vi "Encoder_Correction.vi"(6 "Left X":dbl, 9 "Left Y":dbl, 10 "Right Y":dbl) -> ()   [LabVIEW 2013]
panel:
  out "rr":dbl
  out "fr":dbl
  out "rl":dbl
  out "fl":dbl
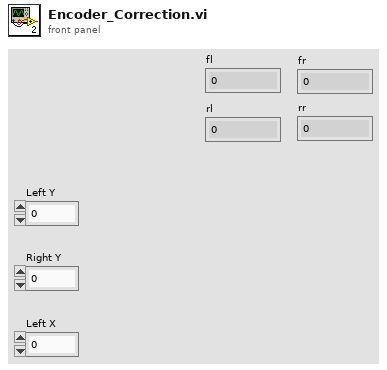
[diagram p1: front panel]
types:
  T1 = typedef "WPI_EncoderDevRef.ctl" = cluster{"DevStatus":errorcluster, "EncoderIndex":T2, "CounterIndex":T3, "DistancePerCount":dbl, "Decoding Type":T4}
  T2 = typedef "FPGA_EncoderIdx.ctl" = enum8{"Enc 0", "Enc 1", "Enc 2", "Enc 3", "Invalid"}
  T3 = typedef "FPGA_CounterCtrSystemIndex.ctl" = enum8{"Ctr 0", "Ctr 1", "Ctr 2", "Ctr 3", "Ctr 4", "Ctr 5", "Ctr 6", "Ctr 7", "Invalid"}
  T4 = typedef "WPI_EncoderType.ctl" = enum16{"1x", "2x", "4x"}
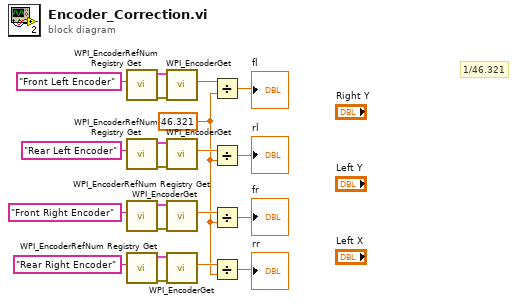
[diagram p0: block diagram]
diagram:
  w1 = 46.321 ("y")
  # "1/46.321"
  n1 = call <vilib>:"WPI_EncoderRefNum Registry Get.vi"("refnum name"="Front Left Encoder") -> ("error out"=w21:errorcluster, "EncoderDevRef"=w20:T1)  [unwired: 9 in]
  n2 = call <vilib>:"WPI_EncoderRefNum Registry Get.vi"("refnum name"="Rear Left Encoder") -> ("error out"=w18:errorcluster, "EncoderDevRef"=w17:T1)  [unwired: 9 in]
  n3 = call <vilib>:"WPI_EncoderRefNum Registry Get.vi"("refnum name"="Front Right Encoder") -> ("error out"=w15:errorcluster, "EncoderDevRef"=w14:T1)  [unwired: 9 in]
  n4 = call <vilib>:"WPI_EncoderRefNum Registry Get.vi"("refnum name"="Rear Right Encoder") -> ("error out"=w12:errorcluster, "EncoderDevRef"=w11:T1)  [unwired: 9 in]
  n5 = call <vilib>:"WPI_EncoderGet.vi"("error in (no error)"=w21, "EncoderDevRef"=w20) -> ("Distance"=w9:dbl)  [unwired: 4 in, 5 out]
  n6 = call <vilib>:"WPI_EncoderGet.vi"("error in (no error)"=w18, "EncoderDevRef"=w17) -> ("Distance"=w8:dbl)  [unwired: 4 in, 5 out]
  n7 = call <vilib>:"WPI_EncoderGet.vi"("error in (no error)"=w15, "EncoderDevRef"=w14) -> ("Distance"=w7:dbl)  [unwired: 4 in, 5 out]
  n8 = call <vilib>:"WPI_EncoderGet.vi"("error in (no error)"=w12, "EncoderDevRef"=w11) -> ("Distance"=w6:dbl)  [unwired: 4 in, 5 out]
  n9 = Divide(x=w9, y=w1) -> (x/y=→"fl":dbl)
  n10 = Divide(x=w8, y=w1) -> (x/y=→"rl":dbl)
  n11 = Divide(x=w7, y=w1) -> (x/y=→"fr":dbl)
  n12 = Divide(x=w6, y=w1) -> (x/y=→"rr":dbl)
